vi "display_3s_stim_3s_ISI_TO1.vi"() -> ()   [LabVIEW 2019]
uses:
  <vilib>/Analysis/Matrix/Datatypes/RealMatrix.ctl
  <vilib>/Utility/file.llb/Write Delimited Spreadsheet (DBL).vi
  <vilib>/Analysis/Matrix/NI_Matrix.lvlib
panel:
  out "Num trials":u32=204
  out "ISI Time":dbl
  out "Stim TS":dbl
  out "Output":dbl[][](array[numeric])
  out "Output frame":T1
  out "Array temp1":T1
  out "Elapsed Time":dbl
  out "Display":bool=TRUE
  out "Trial":u32=1
  out "reward":dbl[](array[numeric])
  out "stim_id":dbl[](array[numeric])
  out "stim_loaded":dbl
  out "Timings":dbl[](array[numeric])
  out "Stimuli Loaded?":bool
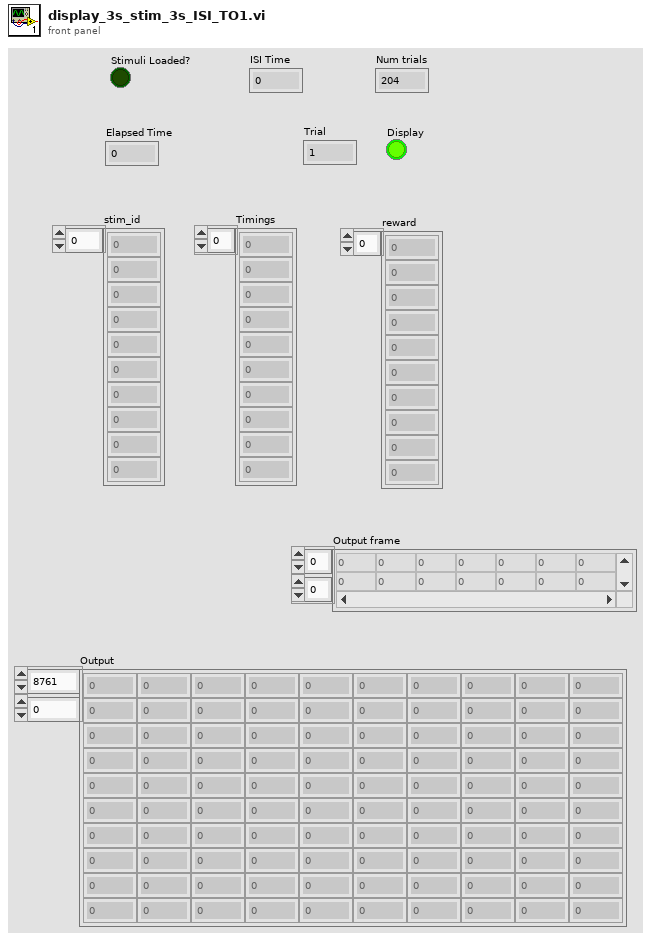
[diagram p1: front panel]
types:
  T1 = typedef "NI_Matrix.lvlib/RealMatrix.ctl" = dbl[][]
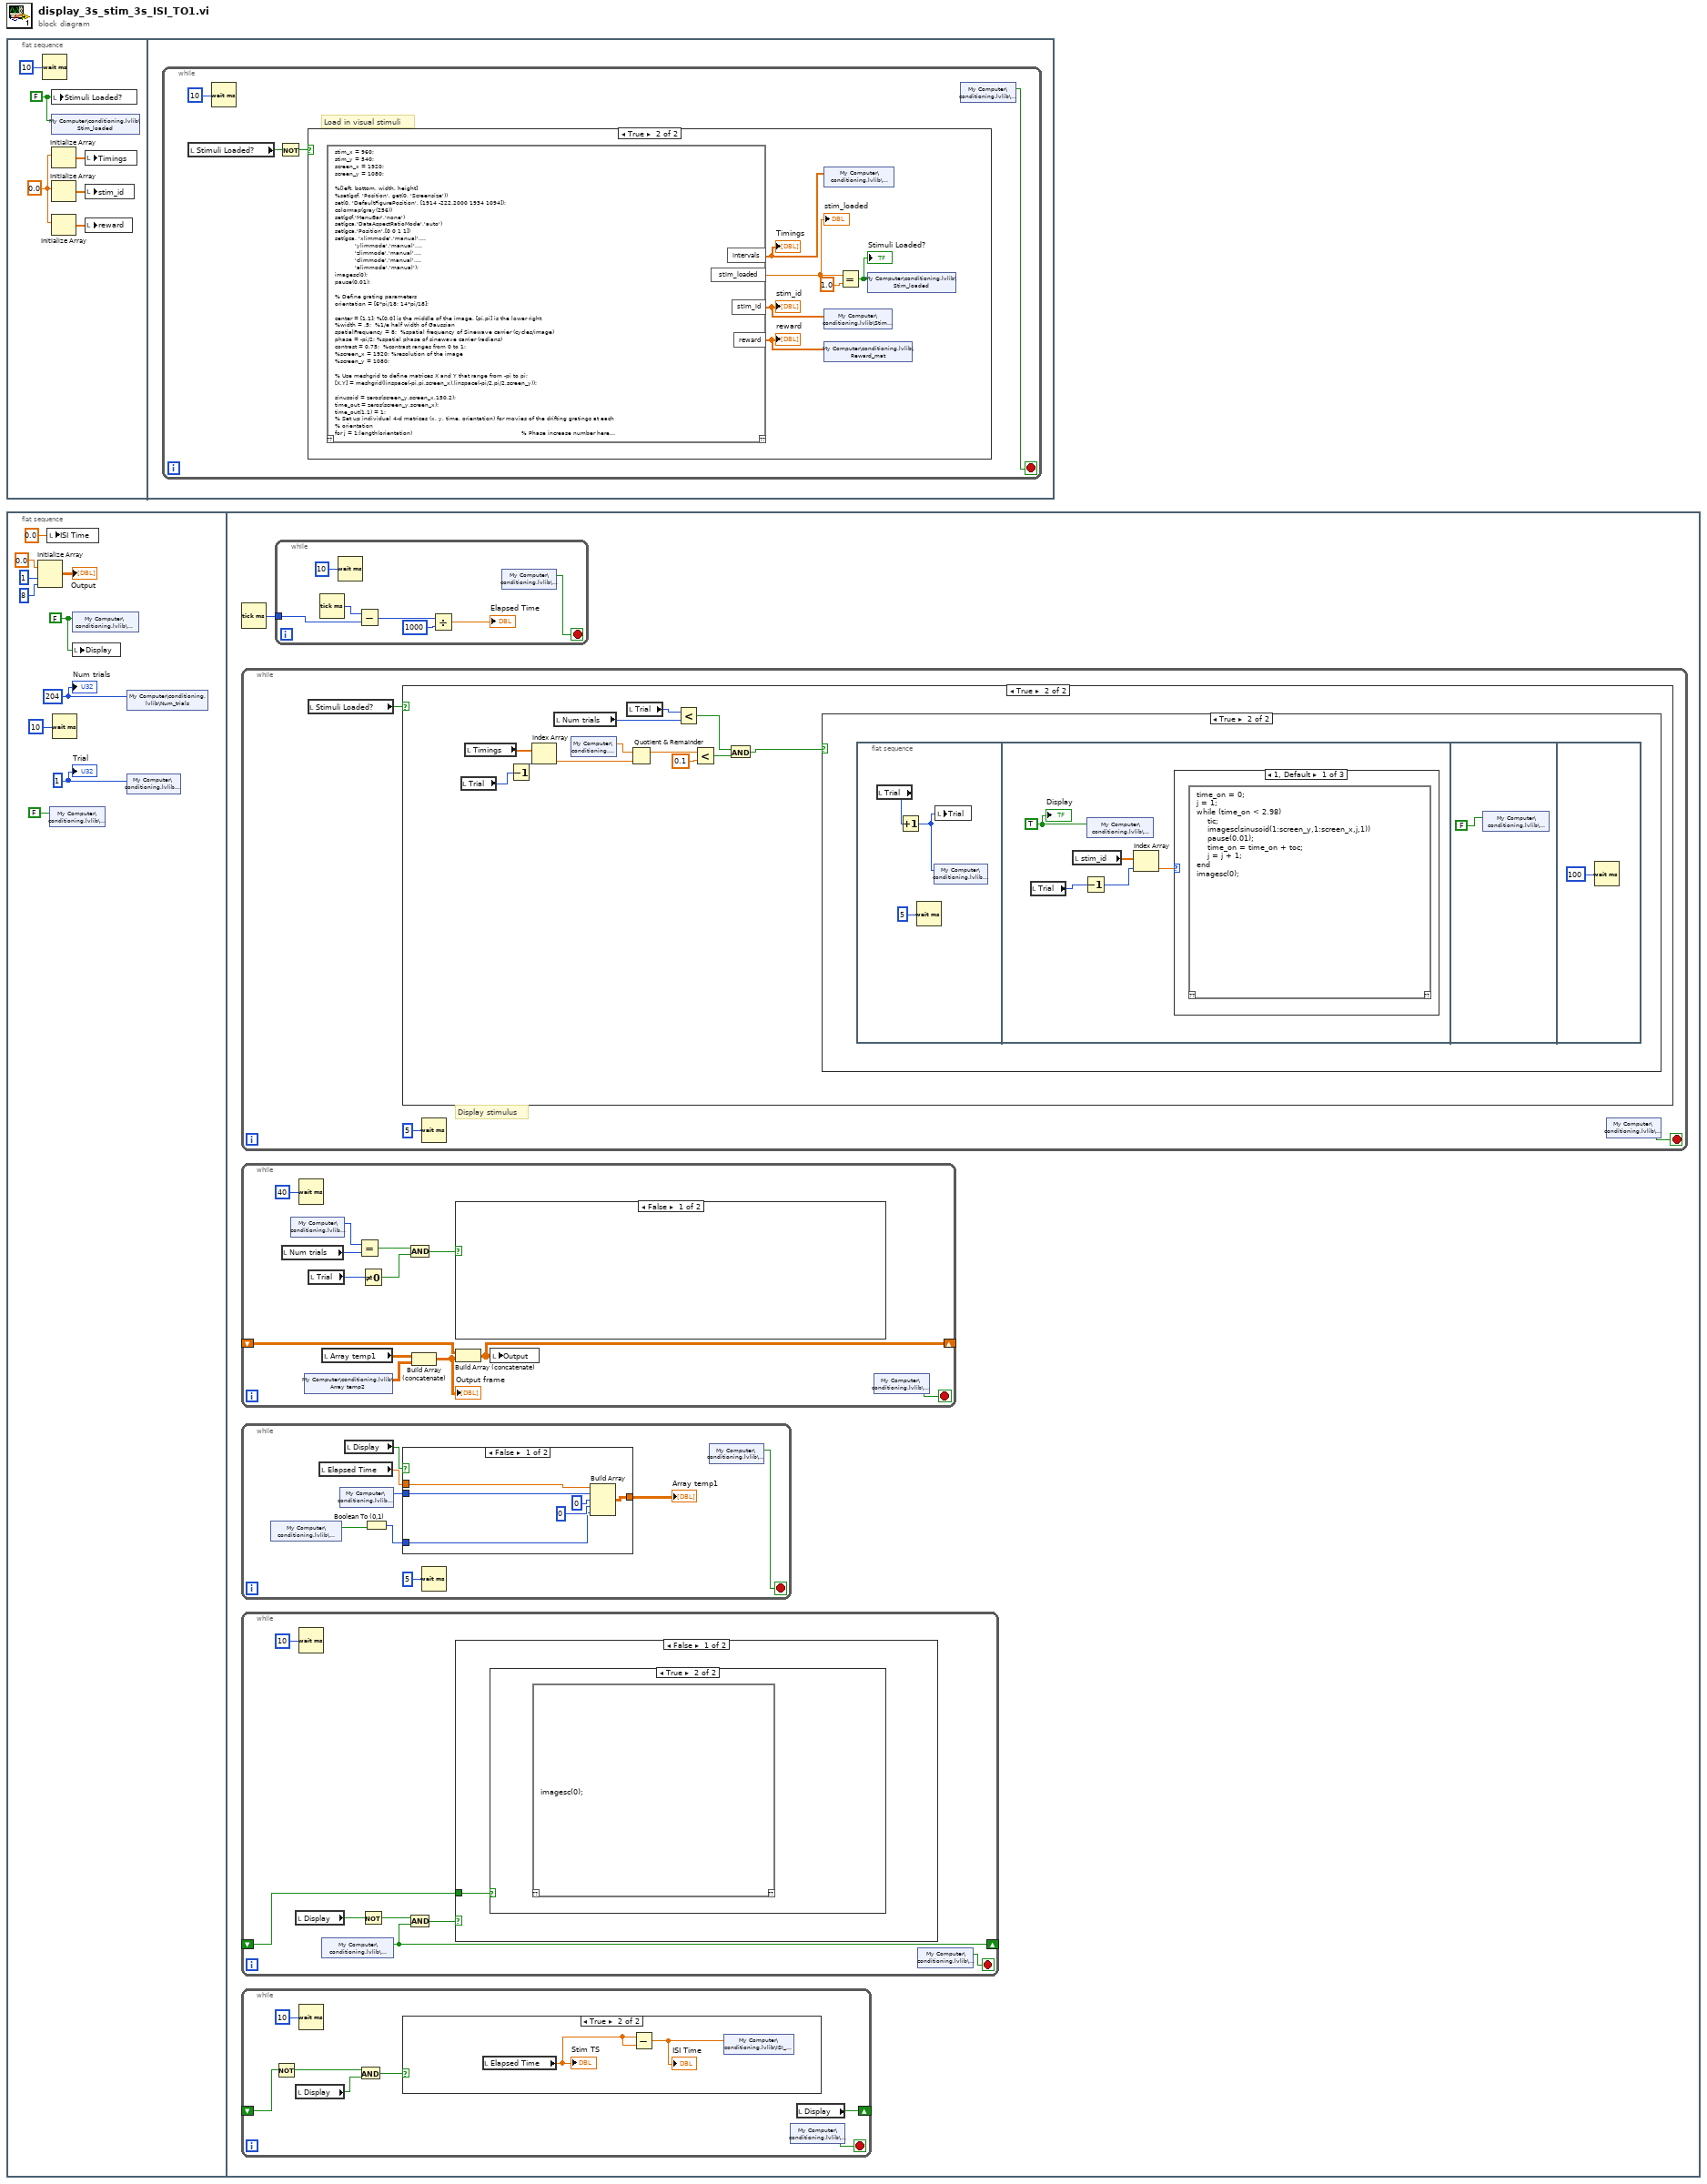
[diagram p0: block diagram]
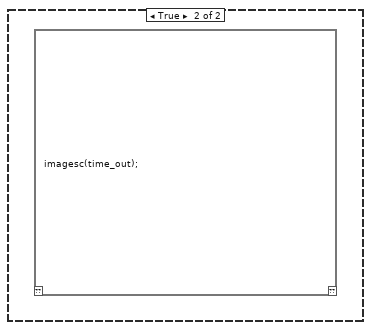
[diagram p4: hidden frame]
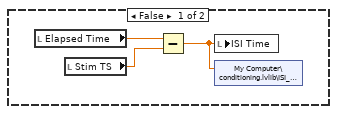
[diagram p5: hidden frame]
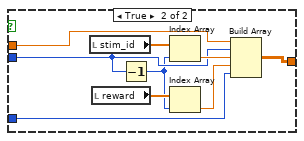
[diagram p6: hidden frame]
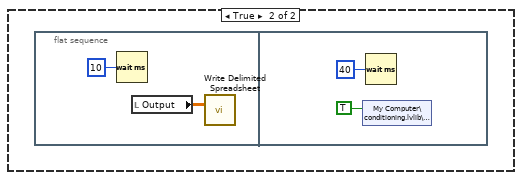
[diagram p7: hidden frame]
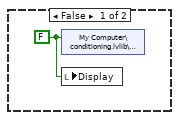
[diagram p9: hidden frame]
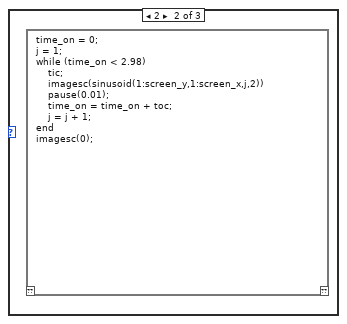
[diagram p10: hidden frame]
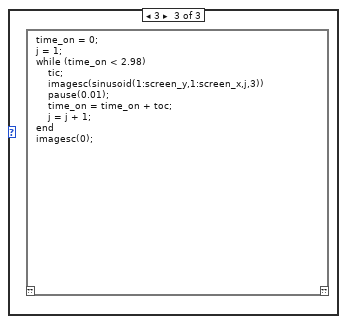
[diagram p11: hidden frame]
diagram:
  n1 = flat-sequence {
    frame #0 {
      w3 = 0.0 ("element")
      w1 = FALSE ("Stimuli Loaded?")
      n2 = Wait (ms)(milliseconds to wait=u32 10) -> ()  [unwired: 1 out]
      n3 = local write "Stimuli Loaded?"(w1) -> ()
      n4 = shared-variable "My Computer\\conditioning.lvlib\\Stim_loaded"(w1) -> ()  [unwired: 1 in, 1 out]
      n5 = Initialize Array(w3) -> (w5:dbl[])  [unwired: 1 in]
      n6 = Initialize Array(w3) -> (w4:dbl[])  [unwired: 1 in]
      n7 = Initialize Array(w3) -> (w2:dbl[])  [unwired: 1 in]
      n8 = local write "Timings"(w5) -> ()
      n9 = local write "stim_id"(w4) -> ()
      n10 = local write "reward"(w2) -> ()
    }
    frame #1 {
      n11 = while {
        stop <- w9 stop-if-true
        # "Load in visual stimuli"
        n12 = local read "Stimuli Loaded?"() -> (w8:bool)
        n13 = Wait (ms)(milliseconds to wait=u32 10) -> ()  [unwired: 1 out]
        n14 = Not(x=w8) -> (.not. x?=w7:bool)
        n15 = case shown="True" w7 {
          frame False {
          }
          frame True {
            n16 = script code="stim_x = 960;\nstim_y = 540;\nscreen_x = 1920;\nscreen_y = 1080;\n\n%[left, bottom, width, height]\n%set(gcf, 'Position', get(0, 'Screensize'))\nset(0, 'DefaultFigurePosition', [1914 -222.2000 1934 1094]);\ncolormap(gray(256))\nset(gcf,'MenuBar','none')\nset(gca,'DataAspectRatioMode','auto')\nset(gca,'Position',[0 0 1 1])\nset(gca, 'xlimmode','manual',...\n           'ylimmode','manual',...\n           'zlimmode','manual',...\n           'climmode','manual',...\n           'alimmode','manual');\nimagesc(0);\npause(0.01);\n\n% Define grating parameters\norientation = [6*pi/18; 14*pi/18];\n\ncenter = [1,1]; %[0,0] is the middle of the image, [pi,pi] is the lower right\n%width = .5;  %1/e half width of Gaussian\nspatialFrequency = 8;  %spatial frequency of Sinewave carrier (cycles/image)\nphase = -pi/2; %spatial phase of sinewave carrier (radians)\ncontrast = 0.75;  %contrast ranges from 0 to 1;\n%screen_x = 1920; %resolution of the image  \n%screen_y = 1080;\n\n% Use meshgrid to define matrices X and Y that range from -pi to pi;\n[X,Y] = meshgrid(linspace(-pi,pi,screen_x),linspace(-pi/2,pi/2,screen_y));\n\nsinusoid = zeros(screen_y,screen_x,150,2);\ntime_out = zeros(screen_y,screen_x);\ntime_out(1,1) = 1;\n% Set up individual 4-d matrices (x, y, time, orientation) for movies of the drifting gratings at each\n% orientation\nfor j = 1:length(orientation)                                                            % Phase increase number here\n    ramp(1:screen_y,1:screen_x,j) = cos(orientation(j))*(X-center(1)) + sin(orientation(j))*(Y-center(2));     %  |\n    for i = 1:150 %Sets the number of frames to define gratings for                   V\n       sinusoid(1:screen_y,1:screen_x,i,j) = contrast*sin(spatialFrequency*ramp(1:screen_y,1:screen_x,j)-...\n           (phase+(2*pi*(i-1)*(-30)/360))); %Number before '/360' sets the phase increase\n    end\nend\n\n%intervals = [ones(1,41)*10 ones(1,41)*11 ones(1,41)*12 ones(1,41)*13 ones(1,40)*14];\nintervals = [ones(1,204)*3];\nstim_id = [ones(1,102)*1 ones(1,102)*2];\n%reward = [ones(1,87)*1 ones(1,15)*0 ones(1,87)*1 ones(1,15)*0];\nreward = [ones(1,204)*1];\n\nrand_idx1 = randperm(204);\nrand_idx2 = randperm(204);\nintervals = intervals(rand_idx2);\nstim_id = stim_id(rand_idx2);\nreward = reward(rand_idx2);\n\nstim_loaded = 1;" ("Script Node")() -> ("stim_loaded"=w16:dbl, "intervals"=w11:dbl[], "stim_id"=w12:dbl[], "reward"=w14:dbl[])  [unwired: 1 in, 1 out]
            "stim_loaded" <- w16
            "Timings" <- w11
            "stim_id" <- w12
            "reward" <- w14
            n17 = shared-variable "My Computer\\conditioning.lvlib\\Timings"(w11) -> ()  [unwired: 1 in, 1 out]
            n18 = shared-variable "My Computer\\conditioning.lvlib\\Stim_ID"(w12) -> ()  [unwired: 1 in, 1 out]
            n19 = shared-variable "My Computer\\conditioning.lvlib\\Reward_mat"(w14) -> ()  [unwired: 1 in, 1 out]
            n20 = Equal?(x=w16, y=1.0) -> (x = y?=w13:bool)
            "Stimuli Loaded?" <- w13
            n21 = shared-variable "My Computer\\conditioning.lvlib\\Stim_loaded"(w13) -> ()  [unwired: 1 in, 1 out]
          }
        }
        n22 = shared-variable "My Computer\\conditioning.lvlib\\Stop"() -> (w9:bool)  [unwired: 1 in, 1 out]
      }
    }
  }
  n23 = flat-sequence {
    frame #0 {
      w18 = u32 204
      w24 = FALSE ("Display")
      w26 = u32 1 ("Trial")
      n24 = Initialize Array(0.0 ("element"), 1 ("dimension size"), 8 ("dimension size")) -> (→"Output":dbl[][])
      n25 = local write "ISI Time"(0.0 ("ISI Time")) -> ()
      n26 = shared-variable "My Computer\\conditioning.lvlib\\Stop"(FALSE ("Stop")) -> ()  [unwired: 1 in, 1 out]
      n27 = Wait (ms)(milliseconds to wait=u32 10) -> ()  [unwired: 1 out]
      n28 = shared-variable "My Computer\\conditioning.lvlib\\Display"(w24) -> ()  [unwired: 1 in, 1 out]
      n29 = local write "Display"(w24) -> ()
      n30 = shared-variable "My Computer\\conditioning.lvlib\\Num_trials"(w18) -> ()  [unwired: 1 in, 1 out]
      n31 = shared-variable "My Computer\\conditioning.lvlib\\Trial"(w26) -> ()  [unwired: 1 in, 1 out]
      "Trial" <- w26
      "Num trials" <- w18
    }
    frame #1 {
      n32 = Tick Count (ms)() -> (millisecond timer value=w27:u32)
      n33 = while {
        stop <- w96 stop-if-true
        # "Display stimulus"
        n34 = local read "Stimuli Loaded?"() -> (w95:bool)
        n35 = case shown="True" w95 {
          frame False {
          }
          frame True {
            n36 = local read "Trial"() -> (w98:u32)
            n37 = local read "Timings"() -> (w107:dbl[])
            n38 = Decrement(x=w98) -> (x-1=w99:u32)
            n39 = Index Array(array=w107, index=w99) -> (element=w106:dbl)
            n40 = local read "Num trials"() -> (w102:u32)
            n41 = shared-variable "My Computer\\conditioning.lvlib\\ISI"() -> (w101:dbl)  [unwired: 1 in, 1 out]
            n42 = local read "Trial"() -> (w105:u32)
            n43 = Quotient & Remainder(x=w101, y=w106) -> (x-y*floor(x/y)=w109:dbl)  [unwired: 1 out]
            n44 = Less?(x=w105, y=w102) -> (x < y?=w104:bool)
            n45 = Less?(x=w109, y=0.1) -> (x < y?=w103:bool)
            n46 = And(x=w104, y=w103) -> (x .and. y?=w100:bool)
            n47 = case shown="True" w100 {
              frame False {
                w110 = FALSE ("Display")
                n48 = shared-variable "My Computer\\conditioning.lvlib\\Display"(w110) -> ()  [unwired: 1 in, 1 out]
                n49 = local write "Display"(w110) -> ()
              }
              frame True {
                n50 = flat-sequence {
                  frame #0 {
                    n51 = local read "Trial"() -> (w113:u32)
                    n52 = Increment(x=w113) -> (x+1=w112:u32)
                    n53 = Wait (ms)(milliseconds to wait=u32 5) -> ()  [unwired: 1 out]
                    n54 = shared-variable "My Computer\\conditioning.lvlib\\Trial"(w112) -> ()  [unwired: 1 in, 1 out]
                    n55 = local write "Trial"(w112) -> ()
                  }
                  frame #1 {
                    w117 = TRUE ("Boolean")
                    n56 = local read "Trial"() -> (w115:u32)
                    n57 = local read "stim_id"() -> (w118:dbl[])
                    n58 = Decrement(x=w115) -> (x-1=w114:u32)
                    n59 = shared-variable "My Computer\\conditioning.lvlib\\Display"(w117) -> ()  [unwired: 1 in, 1 out]
                    n60 = Index Array(array=w118, index=w114) -> (element=w116:dbl)
                    n61 = case shown="1, Default" w116 {
                      frame 1, Default {
                        n62 = script code="time_on = 0;\nj = 1;\nwhile (time_on < 2.98)\n    tic;\n    imagesc(sinusoid(1:screen_y,1:screen_x,j,1))\n    pause(0.01);\n    time_on = time_on + toc;\n    j = j + 1;\nend\nimagesc(0);"() -> ()  [unwired: 1 in, 1 out]
                      }
                      frame 2 {
                        n63 = script code="time_on = 0;\nj = 1;\nwhile (time_on < 2.98)\n    tic;\n    imagesc(sinusoid(1:screen_y,1:screen_x,j,2))\n    pause(0.01);\n    time_on = time_on + toc;\n    j = j + 1;\nend\nimagesc(0);"() -> ()  [unwired: 1 in, 1 out]
                      }
                      frame 3 {
                        n64 = script code="time_on = 0;\nj = 1;\nwhile (time_on < 2.98)\n    tic;\n    imagesc(sinusoid(1:screen_y,1:screen_x,j,3))\n    pause(0.01);\n    time_on = time_on + toc;\n    j = j + 1;\nend\nimagesc(0);"() -> ()  [unwired: 1 in, 1 out]
                      }
                    }
                    "Display" <- w117
                  }
                  frame #2 {
                    n65 = shared-variable "My Computer\\conditioning.lvlib\\Display"(FALSE ("Display")) -> ()  [unwired: 1 in, 1 out]
                  }
                  frame #3 {
                    n66 = Wait (ms)(milliseconds to wait=u32 100) -> ()  [unwired: 1 out]
                  }
                }
              }
            }
          }
        }
        n67 = Wait (ms)(milliseconds to wait=u32 5) -> ()  [unwired: 1 out]
        n68 = shared-variable "My Computer\\conditioning.lvlib\\Stop"() -> (w96:bool)  [unwired: 1 in, 1 out]
      }
      n69 = while {
        shift-right: [w87] -> _
        shift-left: _ -> [w88]
        stop <- w90 stop-if-true
        n70 = local read "Num trials"() -> (w82:u32)
        n71 = shared-variable "My Computer\\conditioning.lvlib\\Trial"() -> (w83:u32)  [unwired: 1 in, 1 out]
        n72 = Wait (ms)(milliseconds to wait=u32 40) -> ()  [unwired: 1 out]
        n73 = shared-variable "My Computer\\conditioning.lvlib\\Array temp2"() -> (w85:dbl[][])  [unwired: 1 in, 1 out]
        n74 = local read "Trial"() -> (w80:u32)
        n75 = local read "Array temp1"() -> (w86:T1)
        n76 = Equal?(x=w83, y=w82) -> (x = y?=w81:bool)
        n77 = Not Equal To 0?(x=w80) -> (x != 0?=w79:bool)
        n78 = And(x=w81, y=w79) -> (x .and. y?=w78:bool)
        n79 = Build Array (concatenate)(w86, w85) -> (w84:T1)
        "Output frame" <- w84
        n80 = case shown="False" w78 {
          frame False {
          }
          frame True {
            n81 = flat-sequence {
              frame #0 {
                n82 = Wait (ms)(milliseconds to wait=u32 10) -> ()  [unwired: 1 out]
                n83 = local read "Output"() -> (w92:dbl[][])
                n84 = call-poly <vilib>:"Write Delimited Spreadsheet.vi"("2D data"=w92) -> ()  [unwired: 13 in, 2 out]
              }
              frame #1 {
                n85 = shared-variable "My Computer\\conditioning.lvlib\\Stop"(TRUE) -> ()  [unwired: 1 in, 1 out]
                n86 = Wait (ms)(milliseconds to wait=u32 40) -> ()  [unwired: 1 out]
              }
            }
          }
        }
        n87 = Build Array (concatenate) ("Build Matrix")(w88, w84) -> (w87:T1)
        n88 = local write "Output"(w87) -> ()
        n89 = shared-variable "My Computer\\conditioning.lvlib\\Stop"() -> (w90:bool)  [unwired: 1 in, 1 out]
      }
      n90 = while {
        stop <- w50 stop-if-true
        n91 = shared-variable "My Computer\\conditioning.lvlib\\Timeout"() -> (w49:bool)  [unwired: 1 in, 1 out]
        n92 = local read "Elapsed Time"() -> (w54:dbl)
        n93 = shared-variable "My Computer\\conditioning.lvlib\\Trial"() -> (w52:u32)  [unwired: 1 in, 1 out]
        n94 = local read "Display"() -> (w51:bool)
        n95 = Boolean To (0,1)(Boolean=w49) -> (0, 1=w48:i16)
        n96 = case shown="False" w51 {
          tunnel: w52 -> [w60 w66]
          tunnel: w54 -> [w61 w68]
          tunnel: [w59 w69] -> w53
          tunnel: w48 -> [w56 w62]
          frame False {
            n97 = Build Array(w61, w60, u32 0 ("milliseconds to wait"), 0, w56) -> (w59:T1)
          }
          frame True {
            n98 = local read "stim_id"() -> (w70:dbl[])
            n99 = local read "reward"() -> (w65:dbl[])
            n100 = Decrement(x=w66) -> (x-1=w64:u32)
            n101 = Index Array(array=w70, index=w64) -> (element=w67:dbl)
            n102 = Index Array(array=w65, index=w64) -> (element=w63:dbl)
            n103 = Build Array(w68, w66, w67, w63, w62) -> (w69:T1)
          }
        }
        "Array temp1" <- w53
        n104 = Wait (ms)(milliseconds to wait=u32 5) -> ()  [unwired: 1 out]
        n105 = shared-variable "My Computer\\conditioning.lvlib\\Stop"() -> (w50:bool)  [unwired: 1 in, 1 out]
      }
      n106 = while {
        shift-right: [w29] -> _
        shift-left: _ -> [w28]
        stop <- w34 stop-if-true
        n107 = local read "Display"() -> (w31:bool)
        n108 = Wait (ms)(milliseconds to wait=u32 10) -> ()  [unwired: 1 out]
        n109 = shared-variable "My Computer\\conditioning.lvlib\\Timeout"() -> (w29:bool)  [unwired: 1 in, 1 out]
        n110 = Not(x=w31) -> (.not. x?=w32:bool)
        n111 = And(x=w32, y=w29) -> (x .and. y?=w30:bool)
        n112 = case shown="False" w30 {
          tunnel: w28 -> [w35 _]
          frame False {
            n113 = case shown="True" w35 {
              frame False {
              }
              frame True {
                n114 = script code="imagesc(0);"() -> ()  [unwired: 1 in, 1 out]
              }
            }
          }
          frame True {
            n115 = script code="imagesc(time_out);"() -> ()  [unwired: 1 in, 1 out]
          }
        }
        n116 = shared-variable "My Computer\\conditioning.lvlib\\Stop"() -> (w34:bool)  [unwired: 1 in, 1 out]
      }
      n117 = while {
        shift-right: [w40] -> _
        shift-left: _ -> [w39]
        stop <- w42 stop-if-true
        n118 = Not(x=w39) -> (.not. x?=w38:bool)
        n119 = local read "Display"() -> (w37:bool)
        n120 = Wait (ms)(milliseconds to wait=u32 10) -> ()  [unwired: 1 out]
        n121 = And(x=w38, y=w37) -> (x .and. y?=w36:bool)
        n122 = case shown="True" w36 {
          frame False {
            n123 = local read "Elapsed Time"() -> (w43:dbl)
            n124 = local read "Stim TS"() -> (w45:dbl)
            n125 = Subtract(x=w43, y=w45) -> (x-y=w44:dbl)
            n126 = local write "ISI Time"(w44) -> ()
            n127 = shared-variable "My Computer\\conditioning.lvlib\\ISI_Time"(w44) -> ()  [unwired: 1 in, 1 out]
          }
          frame True {
            n128 = local read "Elapsed Time"() -> (w46:dbl)
            "Stim TS" <- w46
            n129 = Subtract(x=w46, y=w46) -> (x-y=w47:dbl)
            "ISI Time" <- w47
            n130 = shared-variable "My Computer\\conditioning.lvlib\\ISI_Time"(w47) -> ()  [unwired: 1 in, 1 out]
          }
        }
        n131 = shared-variable "My Computer\\conditioning.lvlib\\Stop"() -> (w42:bool)  [unwired: 1 in, 1 out]
        n132 = local read "Display"() -> (w40:bool)
      }
      n133 = while {
        tunnel: w27 -> [w74]
        stop <- w71 stop-if-true
        n134 = Tick Count (ms)() -> (millisecond timer value=w75:u32)
        n135 = Wait (ms)(milliseconds to wait=u32 10) -> ()  [unwired: 1 out]
        n136 = Subtract(x=w75, y=w74) -> (x-y=w72:u32)
        n137 = Divide(x=w72, y=u32 1000) -> (x/y=→"Elapsed Time":dbl)
        n138 = shared-variable "My Computer\\conditioning.lvlib\\Stop"() -> (w71:bool)  [unwired: 1 in, 1 out]
      }
    }
  }
